vi "Send User Menu Selection.vi"(4 "Item Path":string, 6 "Item Tag":string, 9 "Time":u32, 10 "MenuRef":refnum<k9>, 11 "Message Enqueuer in":refnum<class "Message Enqueuer.lvclass">) -> (0 "error out":errorcluster)   [LabVIEW 2015, in "ActorEvents.lvlib" / "UserMenuSelectionMsg.lvclass"]
doc: "<License>\nCopyright © 2017 Composed Systems, LLC | All rights reserved\nwww.composed.io\n\nAuthor: Ethan Stern <ethan.stern@composed.io>\n\nThis software is provided \"AS IS\" WITHOUT WARRANTIES, either express or implied, AND IS FOR EDUCATIONAL PURPOSES ONLY.\n</License>"
uses:
  UserMenuSelectionMsg.lvclass
  <vilib>/ActorFramework/Message Enqueuer/Message Enqueuer.lvclass
  UserMenuSelectionMsg.lvclass/UserMenuSelectionMsg.ctl
  EventDataMessage/EventDataMessage.lvclass
panel:
  in  "error in (no error)":errorcluster
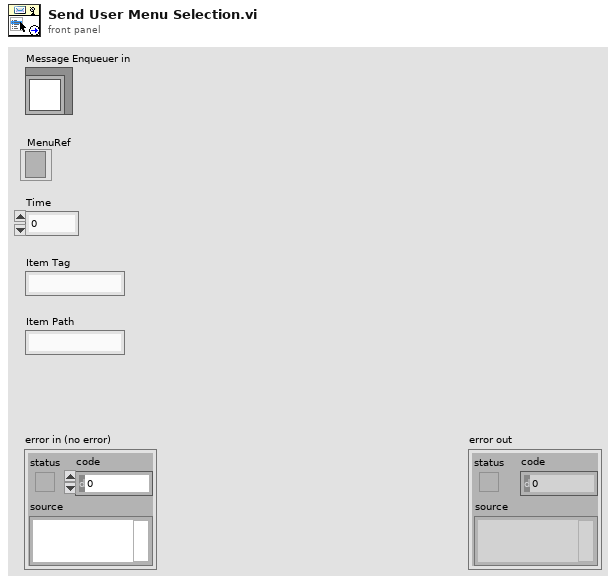
[diagram p1: front panel]
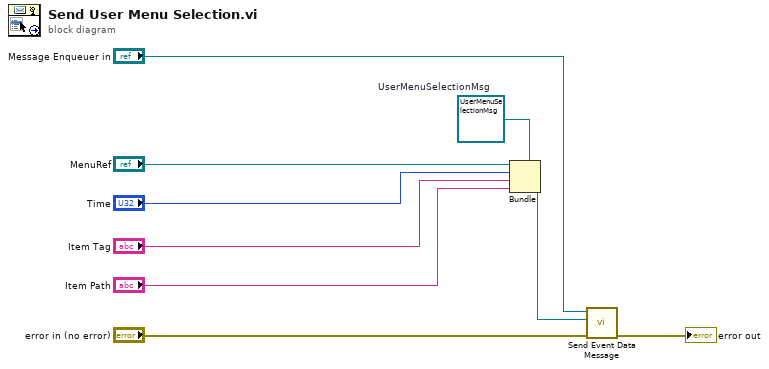
[diagram p0: block diagram]
diagram:
  w9 = refnum<class "UserMenuSelectionMsg.lvclass"> refnum  # UserMenuSelectionMsg
  n1 = Bundle(cluster=w9, "MenuRef", "Time", "Item Tag", "Item Path") -> (w6:refnum<class "UserMenuSelectionMsg.lvclass">)
  n2 = call "Send Event Data Message.vi"("error in (no error)"="error in (no error)", "EventDataMessage in"=w6, "Message Enqueuer in"="Message Enqueuer in") -> ("error out"=→"error out":errorcluster)  [unwired: 8 in]
